vi "7.1-6.7.1-Act Server.vi"() -> ()   [LabVIEW 2010]
doc: "This VI implements a client for the Named Service UDP Server.vi.\nIt connects to a service by specifying the server address and the name of the service. After sending a 'Hello' string to the server, the client receives the string sent by the server, displays the string and closes the connection.\n\n<b>Note:</b> This VI is built to work with the Named Service UDP Server.vi in UDP.llb."
uses:
  7.0-Global.vi
  5-Forebrain/5.7-UDP/5.7 LabVIEW Errors.ctl
  6-OCU Neurons/6.0-Super Heart Beat.ctl
panel:
  in  "error in":errorcluster={"status"=TRUE, "code"=0, "source"=""}
  out "error out":errorcluster
  in  "stop":bool
  out "Probably a hello string":string
  out "Loop Update Cluster":T1
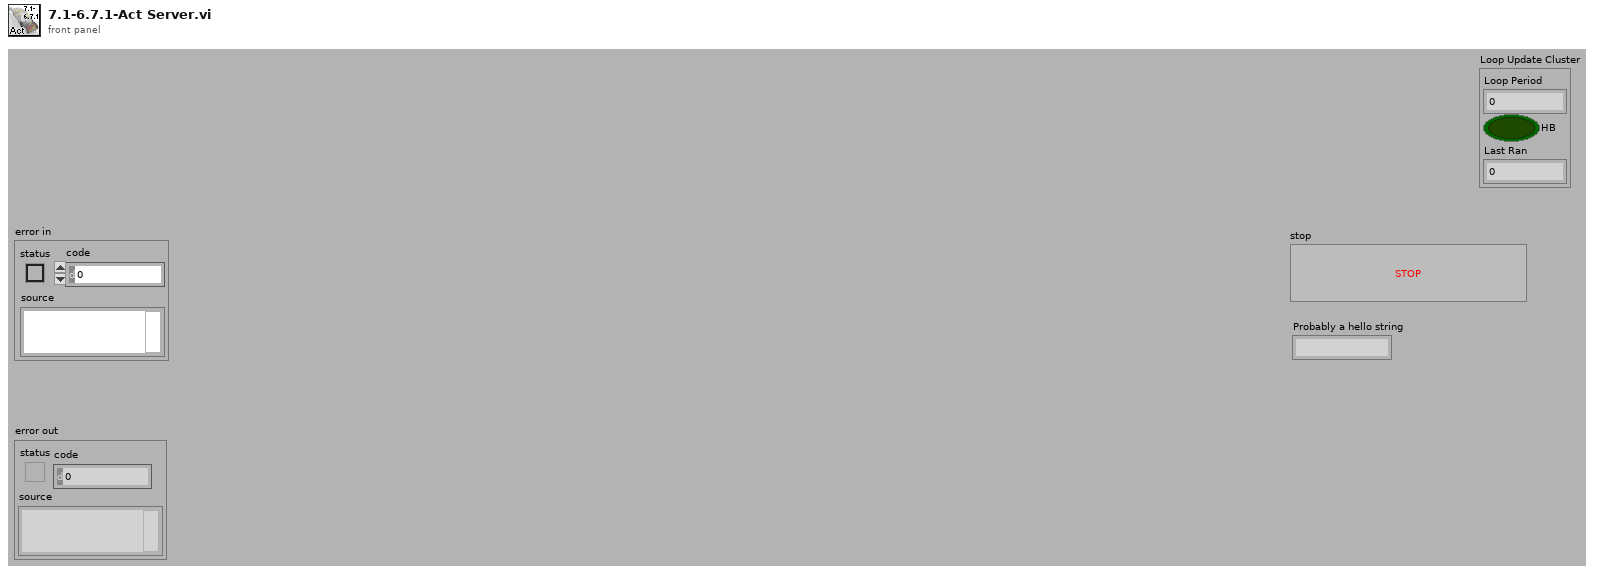
[diagram p1: front panel]
types:
  T1 = typedef "6.0-Super Heart Beat.ctl" = cluster{"Loop Period":u32, "HB":bool, "Last Ran":u32}
  T2 = typedef "6.1-Act.ctl" = cluster{"6.1-Saitek Controller":T3, "Manual Override":bool, "Shutdown":bool, "Reset":bool, "Begin":bool}
  T3 = typedef "6.1-UDP Saitek.ctl" = cluster{"Trig":bool, "2":bool, "3":bool, "4":bool, "5":bool, "6":bool, "7":bool, "8":bool, "9":bool, "10":bool, "11":bool, "Pitch":i32, "Ang":bool[], "Wheel":dbl, "Roll":i32, "Yaw":i32, "Left":i32, "Right":i32}
  T4 = typedef "5.7 LabVIEW Errors.ctl" = i32
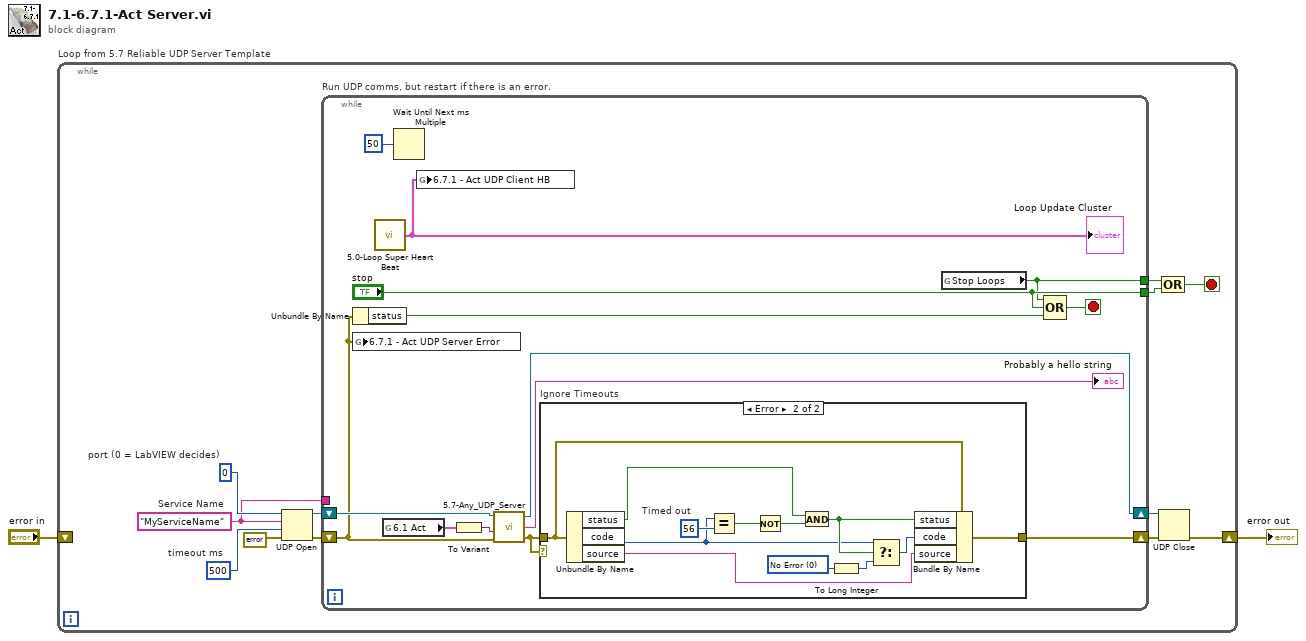
[diagram p0: block diagram]
diagram:
  n1 = while "Loop from 5.7 Reliable UDP Server Template" {
    shift-right: [w7] -> w1
    shift-left: "error in" -> [_]
    stop <- w12 stop-if-true
    w4 = 500  # timeout ms
    w6 = u16 0  # port (0 = LabVIEW decides)
    w5 = "MyServiceName"  # Service Name
    n2 = UDP Open(8:errorcluster {"status"=FALSE, "code"=0, "source"=""} ("error in (no error)"), 9:w4, 10:w5, 11:w6) -> (port=w11:refnum<k16>, 0:w9:errorcluster)  [unwired: 1 in, 1 out]
    n3 = while "Run UDP comms, but restart if there is an error." {
      tunnel: w5 -> [_]
      tunnel: [w17] -> w14
      tunnel: ["stop"] -> w13
      shift-right: [w22] -> w10
      shift-left: w11 -> [w23]
      shift-right: [w24] -> w8
      shift-left: w9 -> [w16]
      stop <- w28 stop-if-true
      n4 = Unbundle By Name(w16) -> ("status"=w25:bool)
      n5 = global write "7.0-Global.vi" "6.7.1 - Act UDP Server Error"(w16) -> ()
      n6 = call "5.0-Loop Super Heart Beat.vi"() -> ("Super Heart Beat"=w15:T1)
      "Loop Update Cluster" <- w15
      n7 = global read "7.0-Global.vi" "6.1 Act"() -> (w18:T2)
      n8 = Wait Until Next ms Multiple(millisecond multiple=u32 50) -> ()  [unwired: 1 out]
      n9 = global write "7.0-Global.vi" "6.7.1 - Act UDP Client HB"(w15) -> ()
      n10 = To Variant(anything=w18) -> (Variant=w21:variant)
      n11 = call "5.7-Any_UDP_Server.vi"("error In"=w16, "Data in"=w21, "Connection ID"=w23) -> ("warning out"=w19:errorcluster, "data out"=→"Probably a hello string":string, "Connection ID out"=w22:refnum<k16>)  [unwired: 1 in]
      n12 = case "Ignore Timeouts" shown="Error" w19 {
        tunnel: w19 -> [w29 w41]
        tunnel: [w29 w40] -> w24
        frame No Error {
        }
        frame Error {
          w31 = T4 0 items=["No Error", "Argument Error", "Memory Full", "Out of Zone", "End of File", "File Already Open", "Generic File IO Error", "File Not Found", "File Permission Error", "Disk Full", "Duplicate Path", "Too Many Files Open", "Not Enabled", "Resource File Not Found", "Cannot Add Resource", "Resource Not Found", "Image Not Found", "Image Memory Error", "Pen Does Not Exist", "Config Bad Type", "Config Token Not Found", "Config Parse Error", "Config Memory Error", "Bad External Code Format", "Bad External Code Offset", "External Code Not Present", "Null Window", "Destroy Window Mixup", "Null Menu", "Print Aborted", "Bad Print Record", "Print Driver Error", "Windows Error During Print", "Memory Error During Print", "Print Dialog Error", "Generic Print Error", "Invalid Device Refnum", "Device Not Found", "Device Parameter Error", "Device Unit Error", "Can't Open Device", "Device Call Aborted", "Generic Error", "Cancelled By User", "Object ID Too Low", "Object ID Too High", "Object Not In Heap", "Unknown Heap", "Bad DefProc ID", "DefProc Not In Table", "Message Out Of Range", "Null Method", "Unknown Message", "Manager Call Not Supported", "Bad address", "Connection In progress", "Connection timed out", "Connection is already in progress", "Network attribute not supported", "Network error", "Address in use", "System out of memory", "Connection aborted", "Connection refused", "Connection is not connected", "Connection is already connected", "Connection closed", "Initialize error (interapplication manager)", "Bad occurrence", "Wait on unbound occurrence handler", "Occurrence queue overflow", "Bad path", "Semaphore not signaled", "Unrecognized type (interapplication manager)"] ("1st Error to Convert")
          w39 = 56  # Timed out
          n13 = Unbundle By Name(w41) -> ("status"=w36:bool, "code"=w34:i32, "source"=w32:string)
          n14 = Equal?(x=w34, y=w39) -> (x = y?=w38:bool)
          n15 = Not(x=w38) -> (.not. x?=w37:bool)
          n16 = And(x=w36, y=w37) -> (x .and. y?=w35:bool)
          n17 = To Long Integer(number=w31) -> (32bit integer=w30:T4)
          n18 = Select(t=w34, s=w35, f=w30) -> (s? t:f=w33:T4)
          n19 = Bundle By Name(cluster=w41, "status"=w35, "code"=w33, "source"=w32) -> (w40:errorcluster)
        }
      }
      n20 = global read "7.0-Global.vi" "Stop Loops"() -> (w17:bool)
      n21 = Compound Arithmetic op=OR(w17, "stop", w25) -> (w28:bool)
    }
    n22 = UDP Close(connection ID=w10, 8:w8) -> (error out=w7:errorcluster)  [unwired: 1 out]
    n23 = Compound Arithmetic op=OR(w14, w13) -> (w12:bool)
  }
  "error out" <- w1
